vi "A Syringe Run.vi"() -> ()   [LabVIEW 2010]
panel:
  out "Accumulated Volume (ul)":dbl format="%#_6f"
  out "Flow Rate (ul/min)":dbl format="%#_6f"
  out "force setting (0-100)":dbl format="%#_6f"
  out "Diameter (mm)":dbl format="%#_6f"
  in  "Flow Rate (ul/min)  2":dbl=20.0
  in  "Force (1-100)":dbl=100.0
  in  "Diameter (mm)   2":dbl=10.0
  in  "stop":bool
  out "Run":bool
  in  "32 -> slow\n31 -> fast":refnum<visa-resource-name>="COM18"
  # "Syringe Pump Values"
  # "Syringe Pump Inputs"
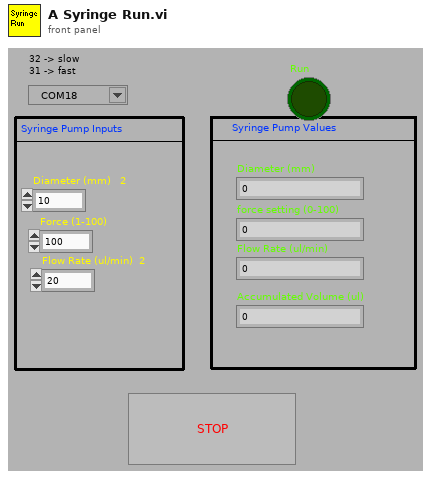
[diagram p1: front panel]
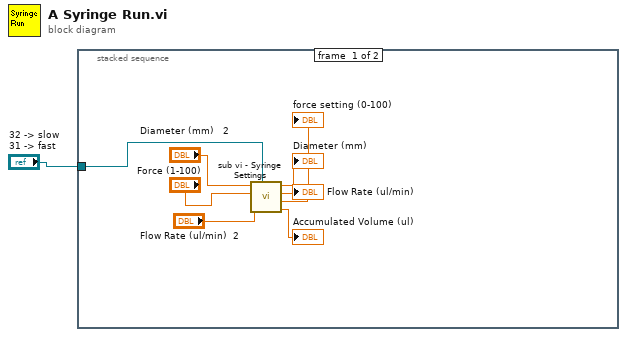
[diagram p0: block diagram]
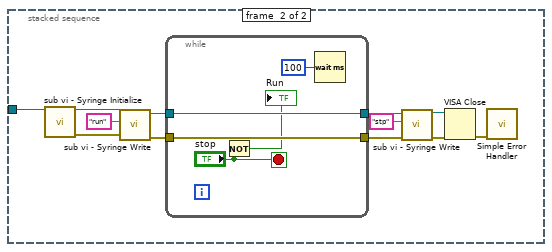
[diagram p2: hidden frame]
diagram:
  n1 = stacked-sequence {
    tunnel: "32 -> slow\n31 -> fast" -> [w2 w21]
    frame #0 {
      n2 = call "sub vi - Syringe Settings.vi"("VISA resource name"=w2, "Flow Rate (ul/min)"="Flow Rate (ul/min)  2", "Force (1-100)"="Force (1-100)", "Diameter (mm)"="Diameter (mm)   2") -> ("Accumulated Volume (ul)"=→"Accumulated Volume (ul)":dbl, "Flow Rate (ul/min)"=→"Flow Rate (ul/min)":dbl, "force setting (0-100)"=→"force setting (0-100)":dbl, "Diameter (mm)"=→"Diameter (mm)":dbl)  [unwired: 4 out]
    }
    frame #1 {
      n3 = call "sub vi - Syringe Initialize.vi"("VISA resource name"=w21) -> ("VISA resource name out"=w20:refnum<visa-resource-name>, "error out"=w19:errorcluster)  [unwired: 13 out]
      n4 = call "sub vi - Syringe Write.vi"("error out"=w19, "Command"="run", "VISA resource name out"=w20) -> ("error out 2"=w16:errorcluster, "VISA resource name out 2"=w17:refnum<visa-resource-name>)  [unwired: 7 out]
      n5 = while {
        tunnel: w17 -> [w26]
        tunnel: w16 -> [w25]
        tunnel: [w26] -> w10
        tunnel: [w25] -> w11
        stop <- "stop" stop-if-true
        n6 = Not(x="stop") -> (.not. x?=→"Run":bool)
        n7 = Wait (ms)(milliseconds to wait=u32 100) -> ()  [unwired: 1 out]
      }
      n8 = call "sub vi - Syringe Write.vi"("error out"=w11, "Command"="stp", "VISA resource name out"=w10) -> ("error out 2"=w13:errorcluster, "VISA resource name out 2"=w12:refnum<visa-resource-name>)  [unwired: 7 out]
      n9 = VISA Close(VISA resource name=w12, error in (no error)=w13) -> (error out=w14:errorcluster)
      n10 = call <vilib>:"Simple Error Handler.vi"("error in (no error)"=w14) -> ()  [unwired: 1 in, 8 out]
    }
  }
